vi "ResultsDB Select data.vi"(7 "CMD":T1(ring), 8 "error in (no error)":errorcluster, 9 "ItemsID":string, 11 "MainBarcode":string) -> (0 "error out":errorcluster, 2 "File Paht":string[](array[string]), 3 "30 rows":string[][](array[string]))   [LabVIEW 2015]
doc: "开始测试时根据条目自动创建条目条目，生产文件路径。\n#2020-6-8 13:25:45"
uses:
  SQLite.lvclass
  <userlib>/LabSQL/LabSQL.lvlib
  <userlib>/sushu/sushu.lvlib
  vi.lib/TopPath.lvlib
panel:
  out "32bit integer":i32
  out "size(s)":i32
  out "String":string
  out "Update CMD":string
  out "element":string
  out "Table Control":string[][](table)
  out "resulting string":string
  out "CMD":string
  out "error out 2":errorcluster
  out "match substring":string
  out "number (0 to 1)":dbl
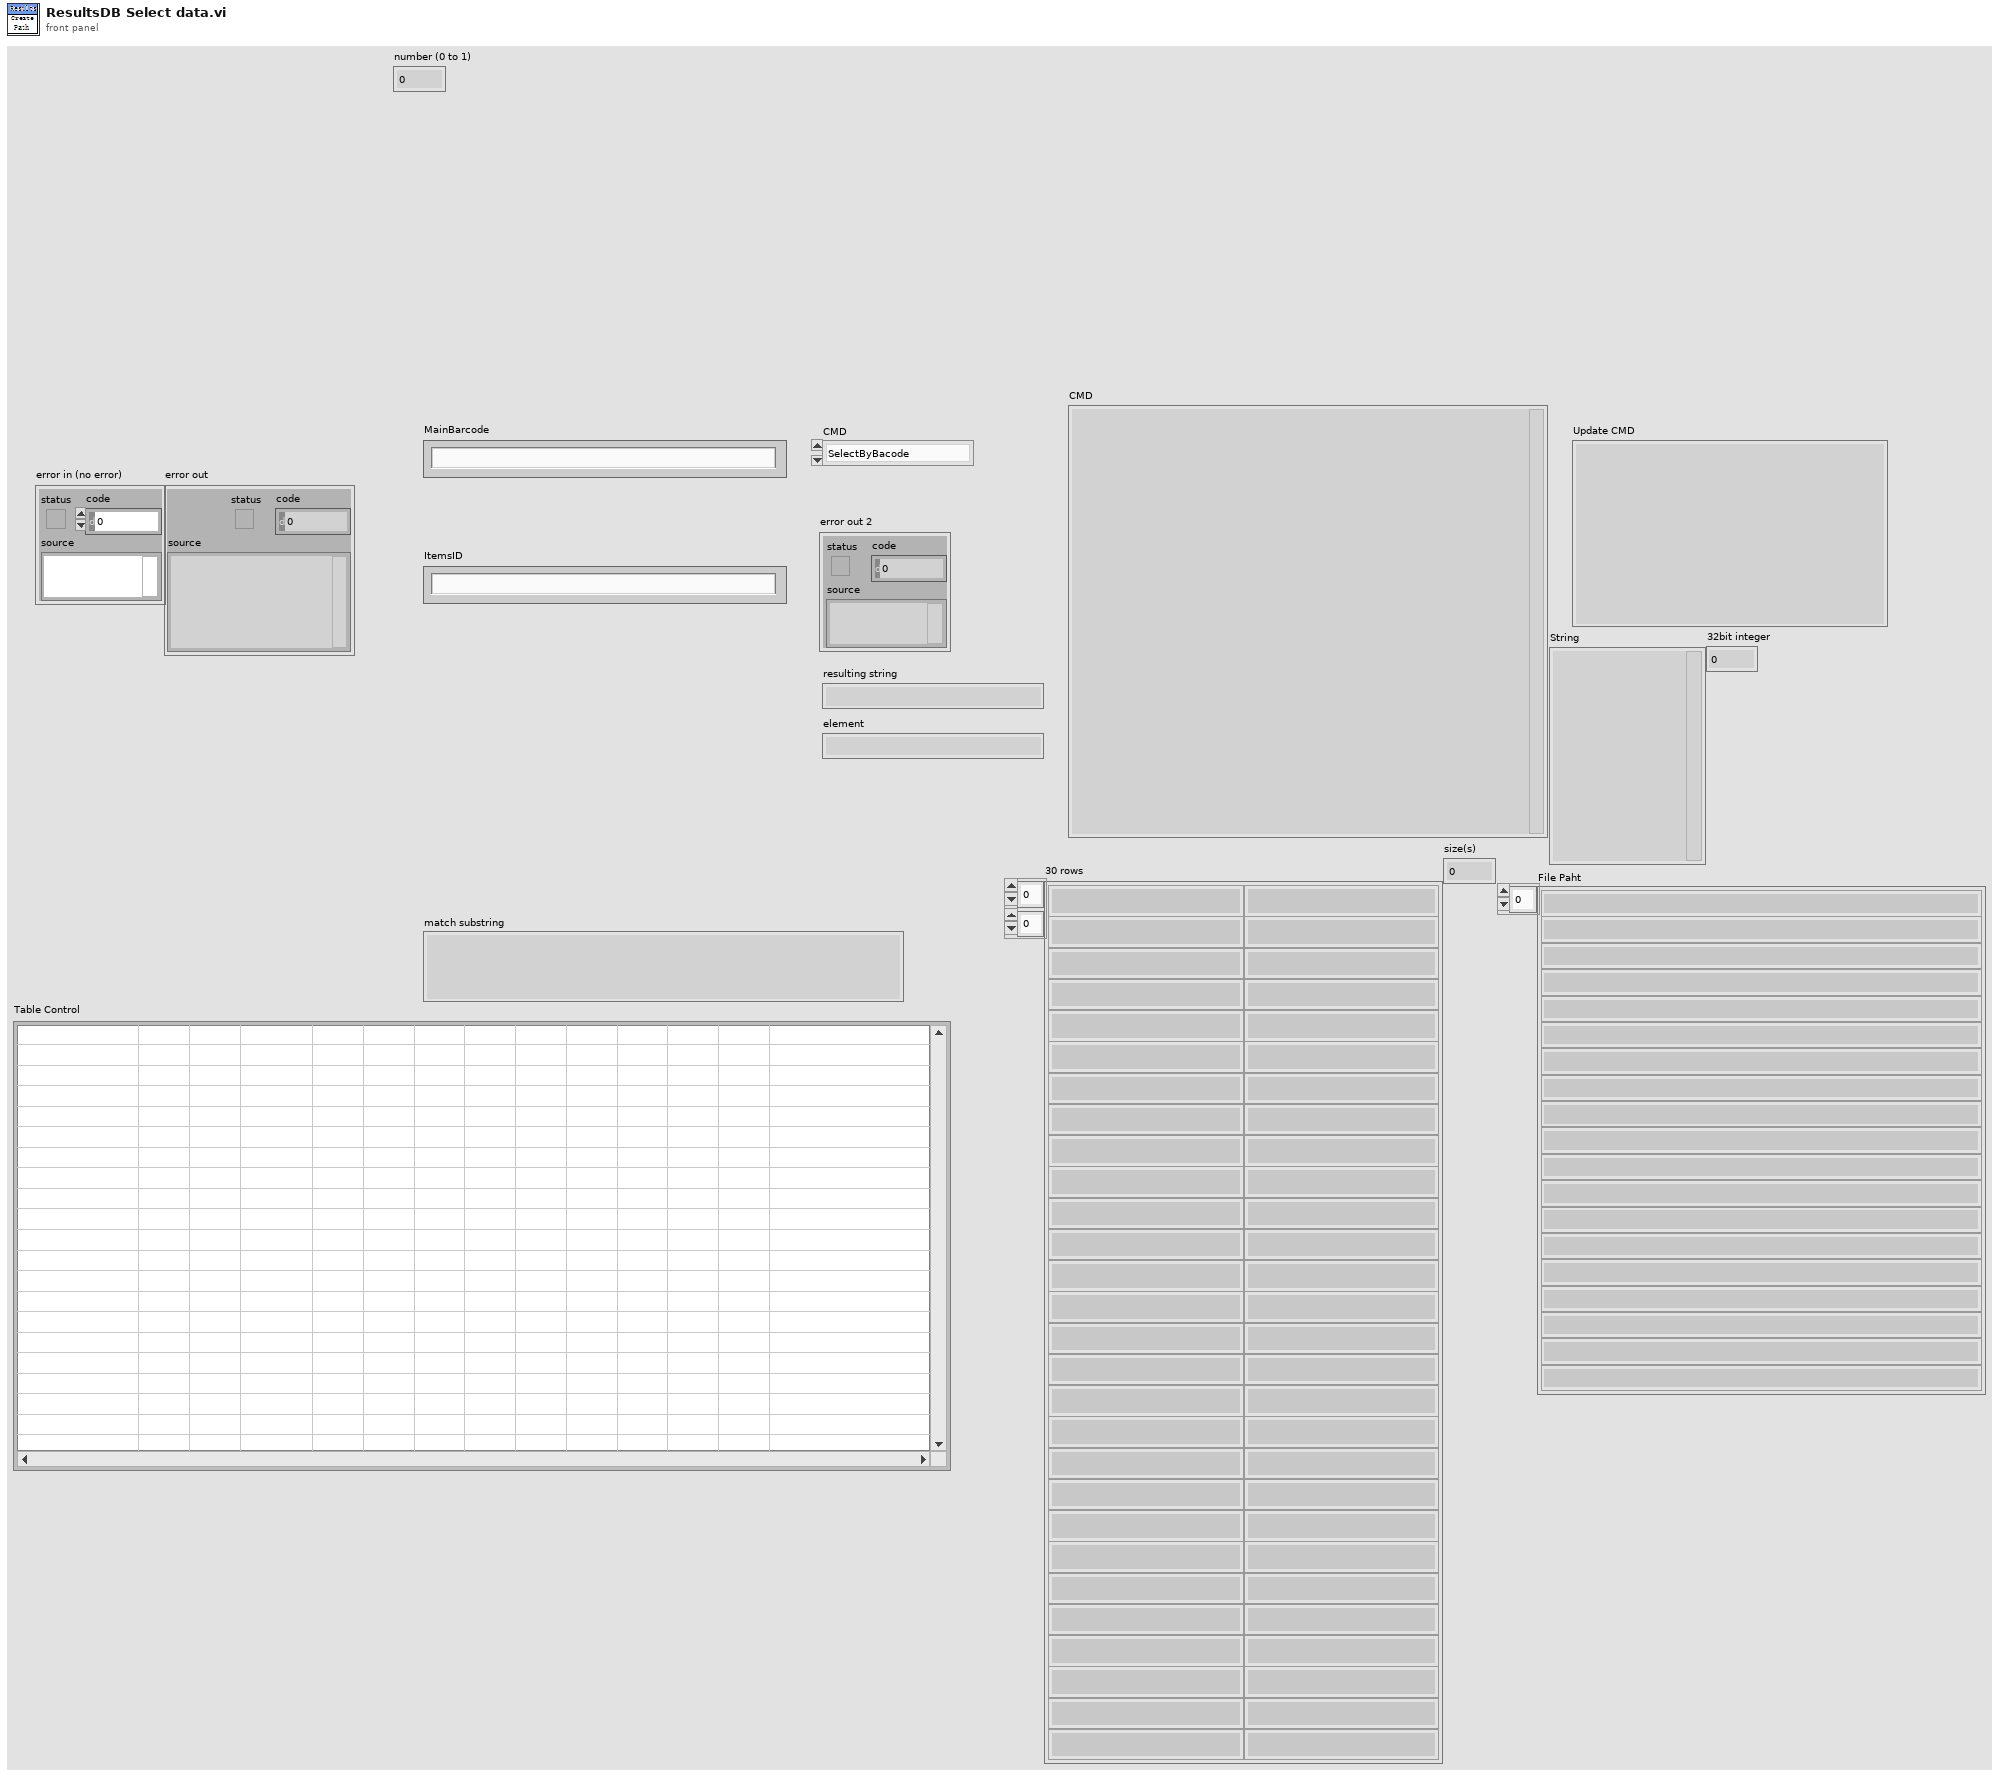
[diagram p1: front panel]
types:
  T1 = enum16{"SelectByBacode", "SelectByDatetime", "Update-UploadColumn"}
  T2 = cluster{"Core":cluster{"Current VI Reference":refnum<vi>, "Close Panel on Exit?":bool}, "VI Name":string, "Row Numbers":string, "Update?":bool, "Results Folder path":path, "CMD":string, "RowNum":i32, "ResultFilePath":path, "InsertTimes":i32}
  T3 = typedef "sushu_vi_lib.lvlib/TopPath.lvlib/Top Path.ctl" = cluster{"LV Source":path, "FilePath":path, "Data":path}
  T4 = enum16{"Other", "SQL2008", "SQLite", "Access", "MySQL"}
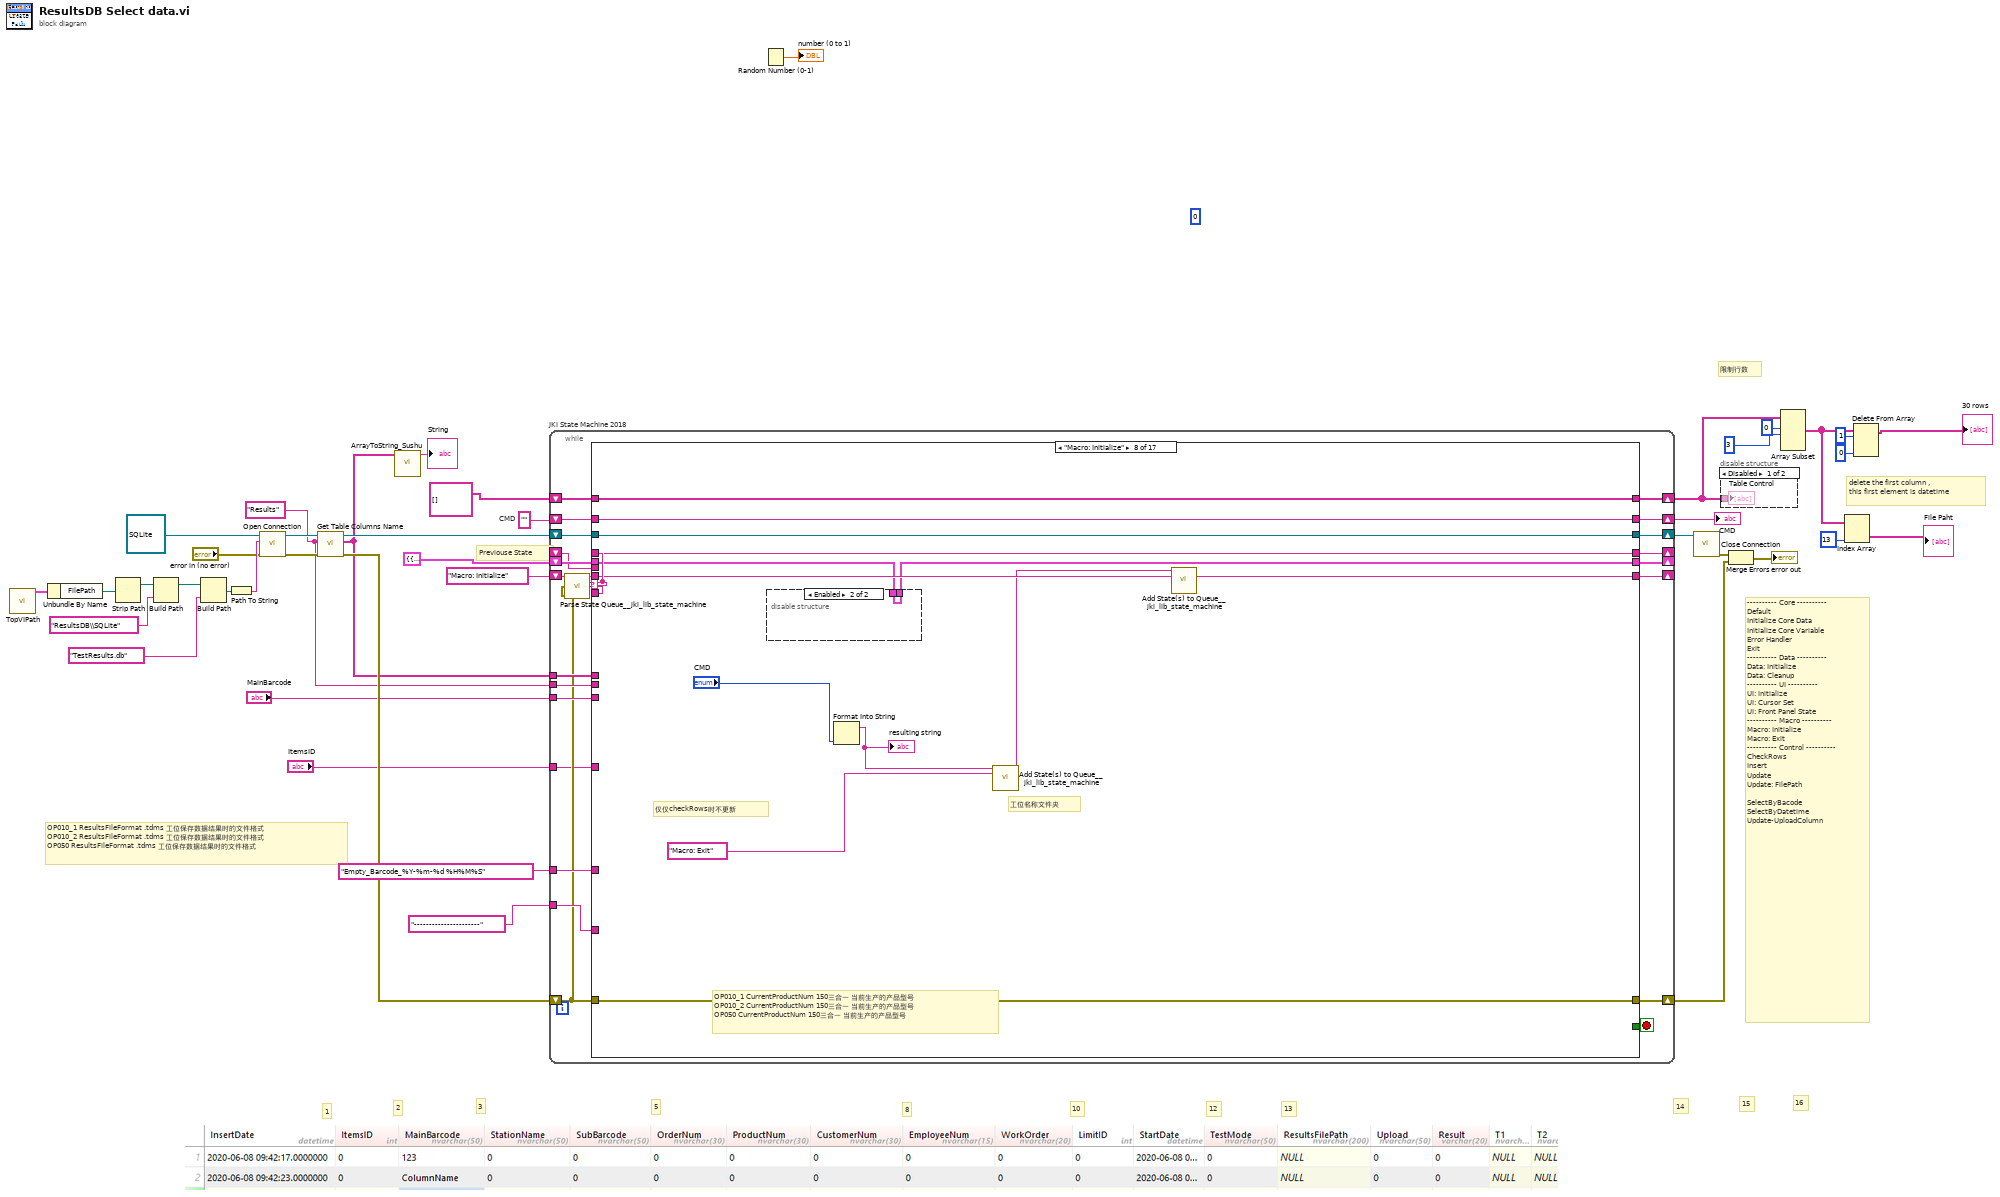
[diagram p0: block diagram]
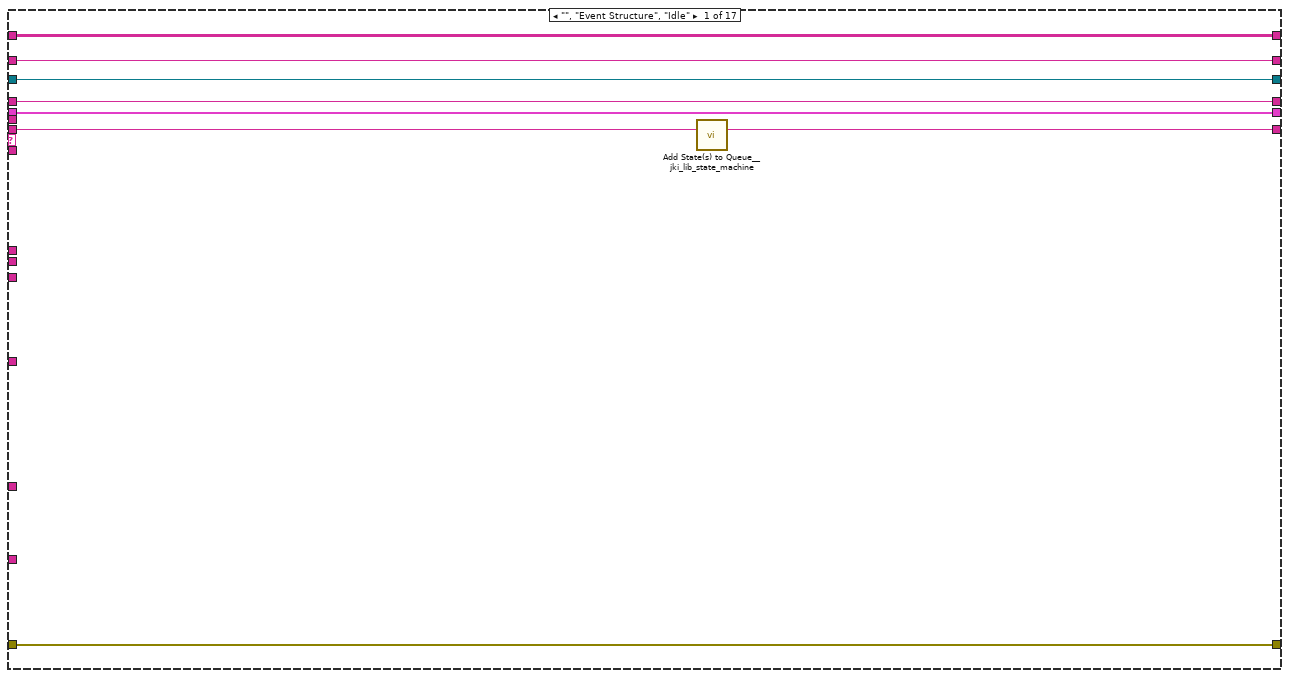
[diagram p3: hidden frame]
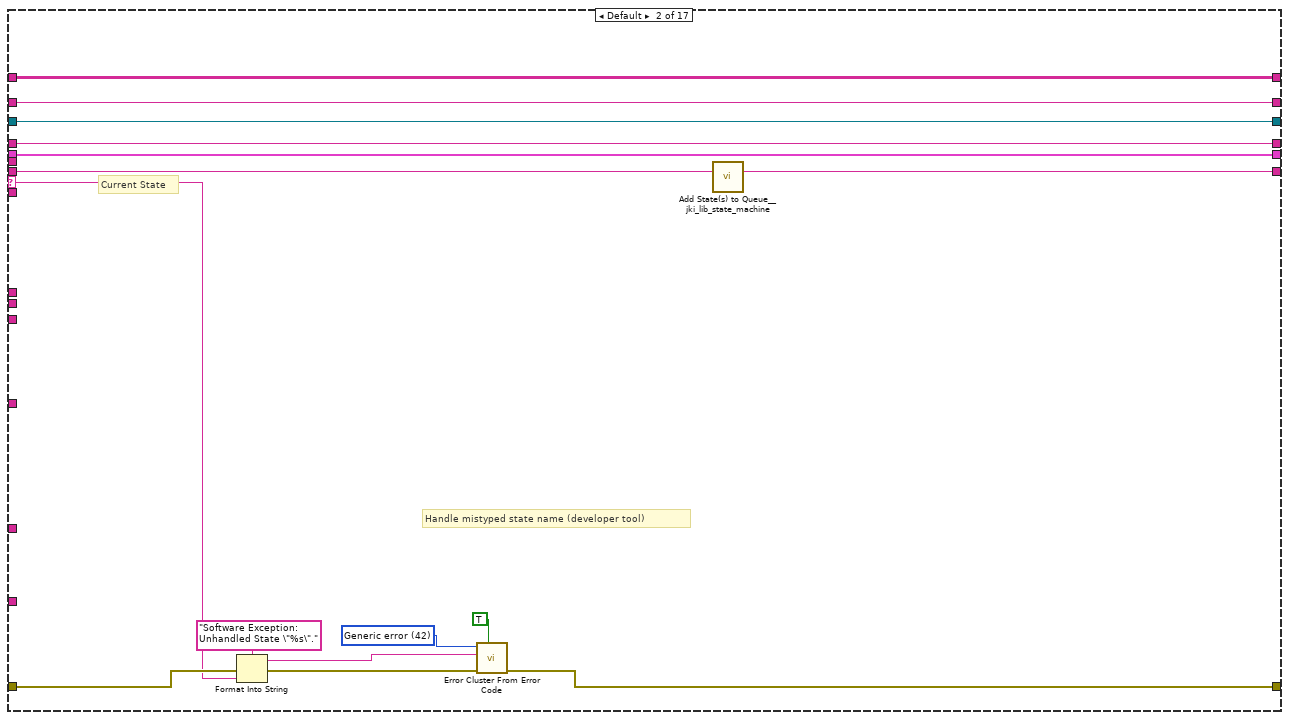
[diagram p4: hidden frame]
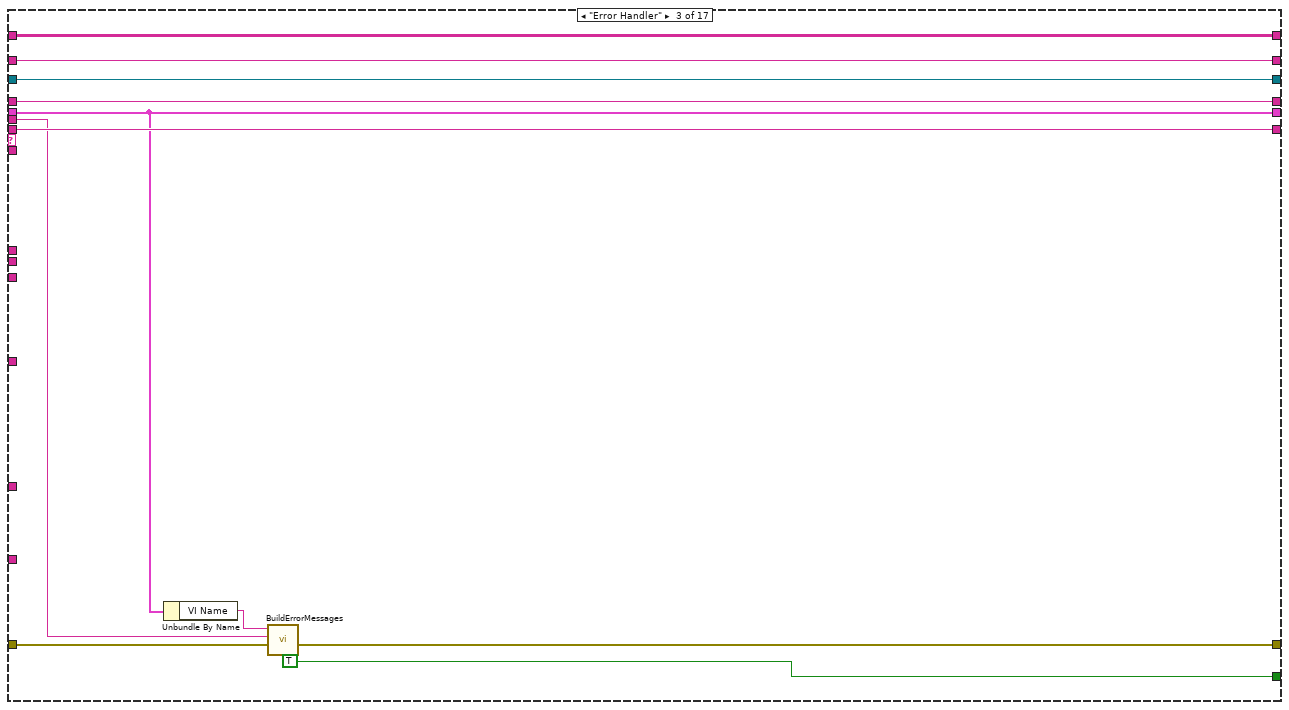
[diagram p5: hidden frame]
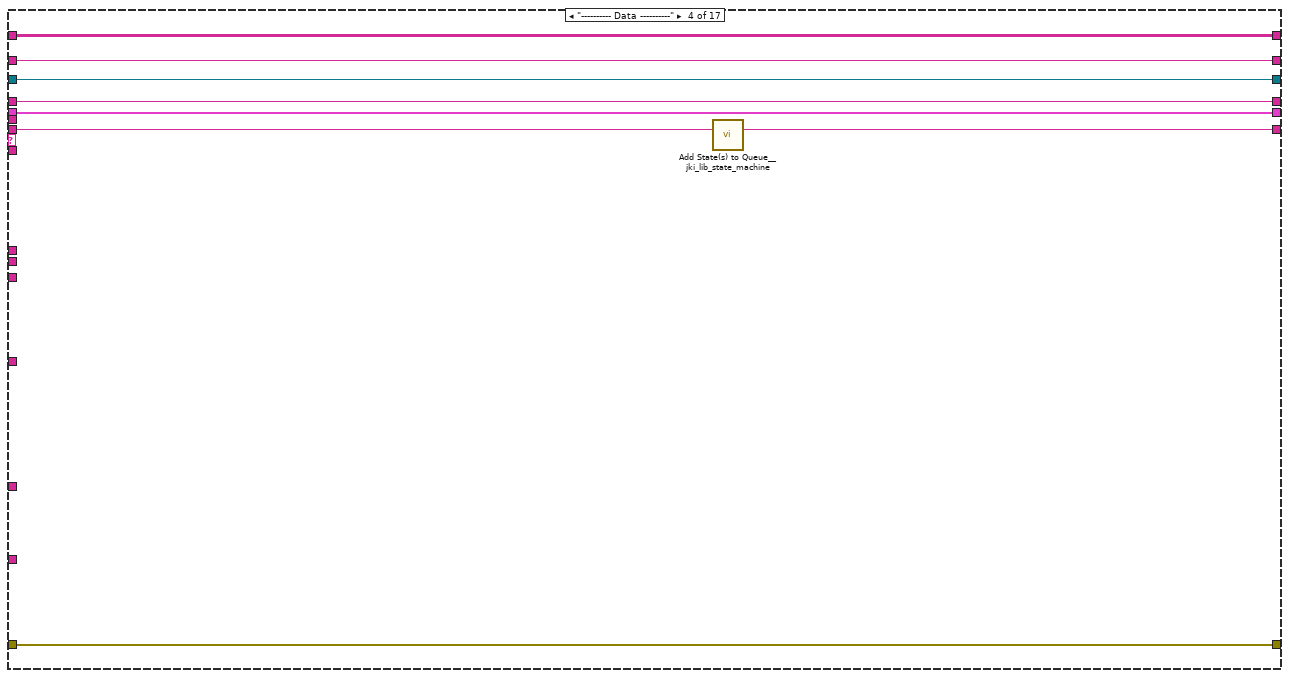
[diagram p6: hidden frame]
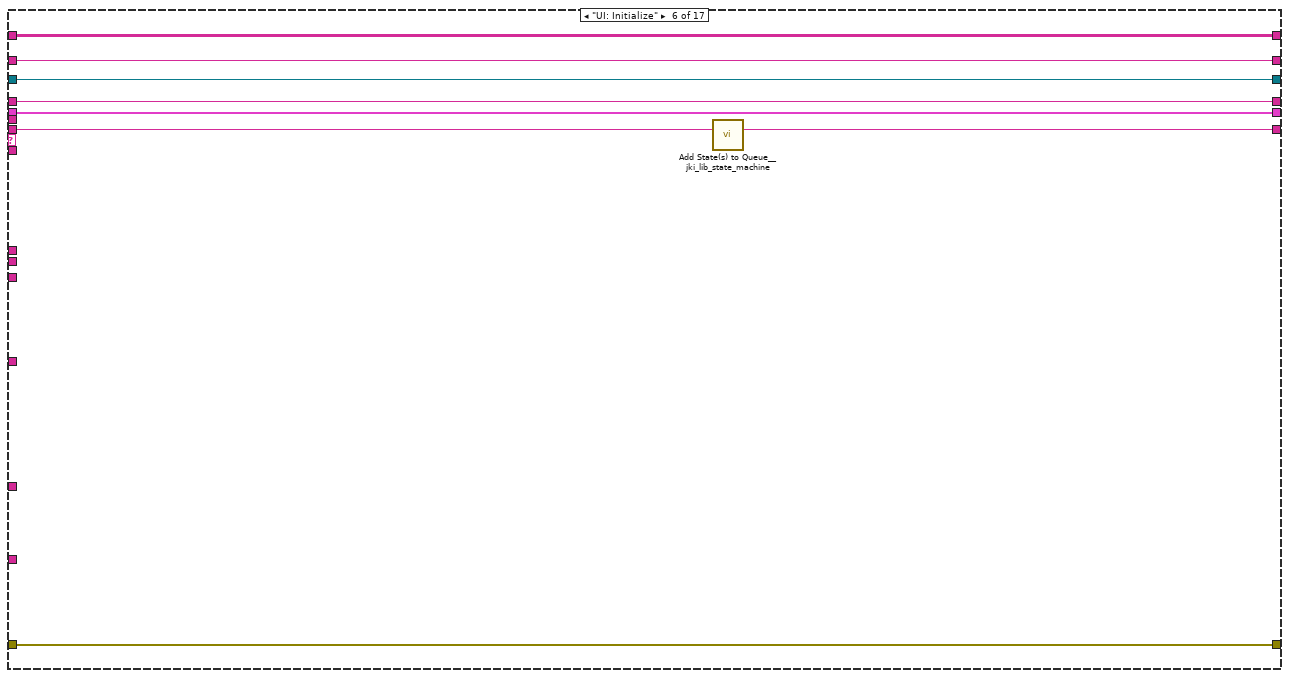
[diagram p8: hidden frame]
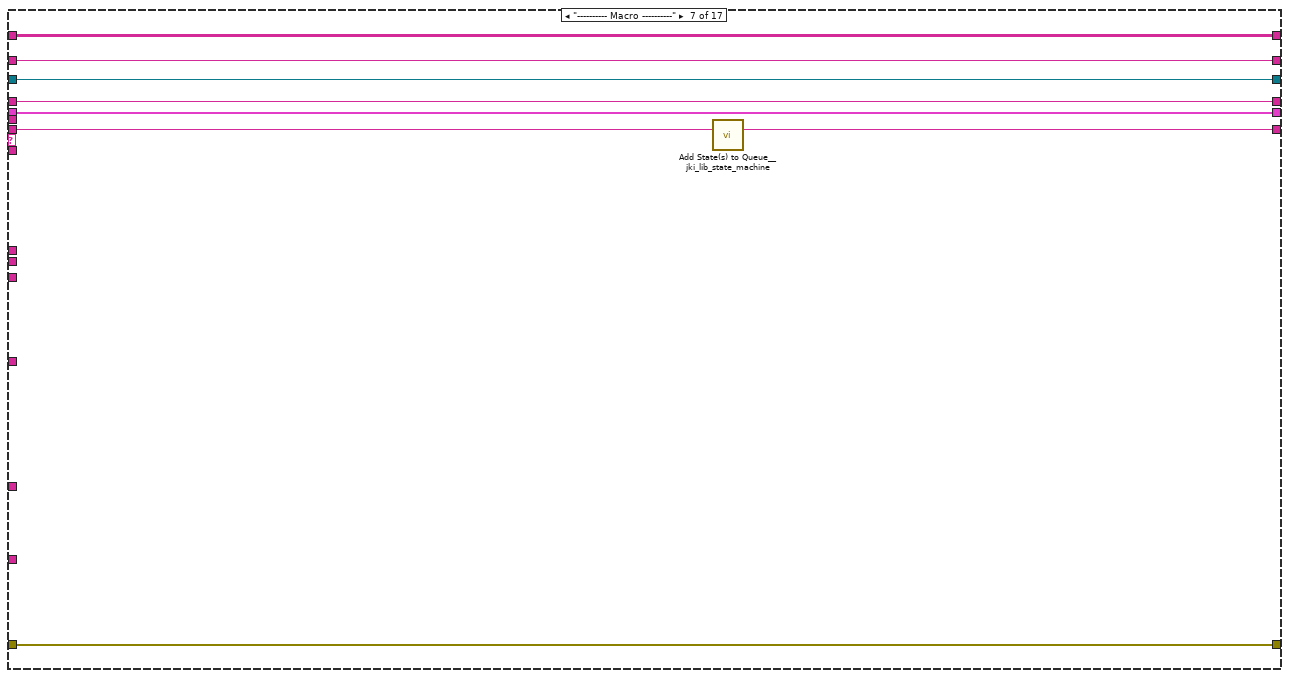
[diagram p9: hidden frame]
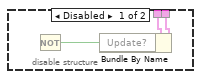
[diagram p10: hidden frame]
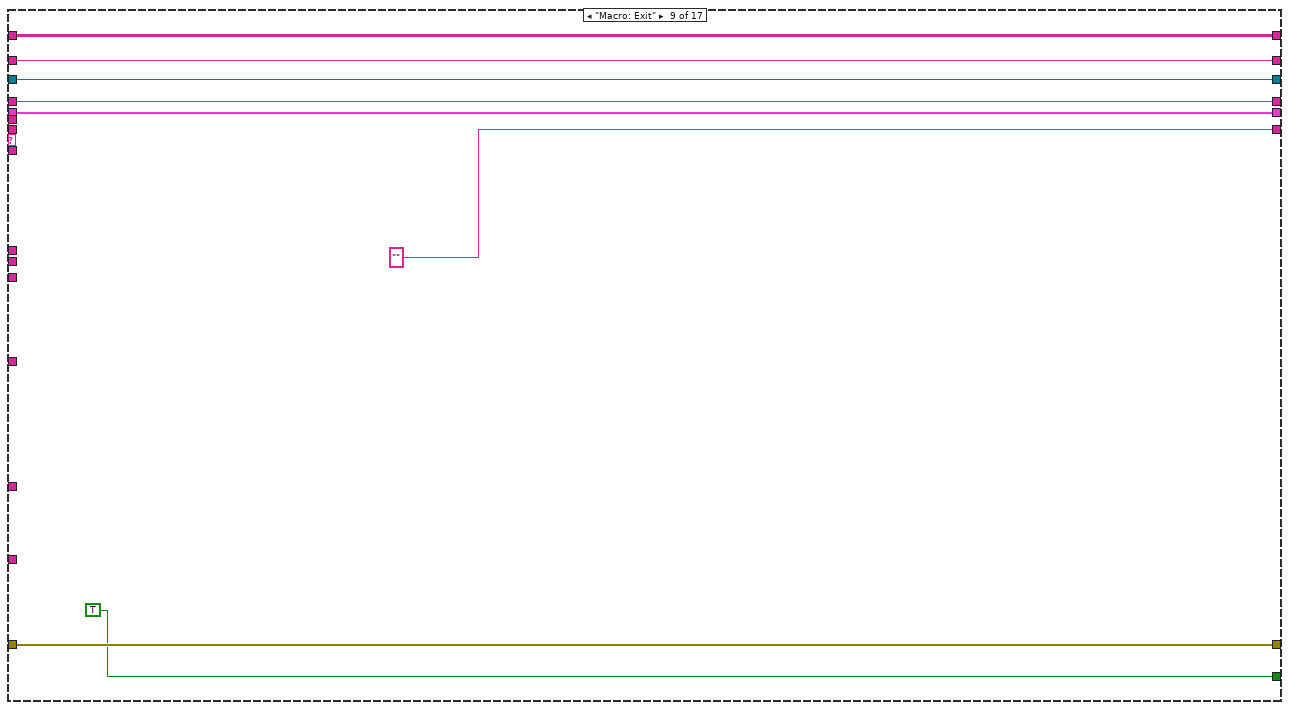
[diagram p11: hidden frame]
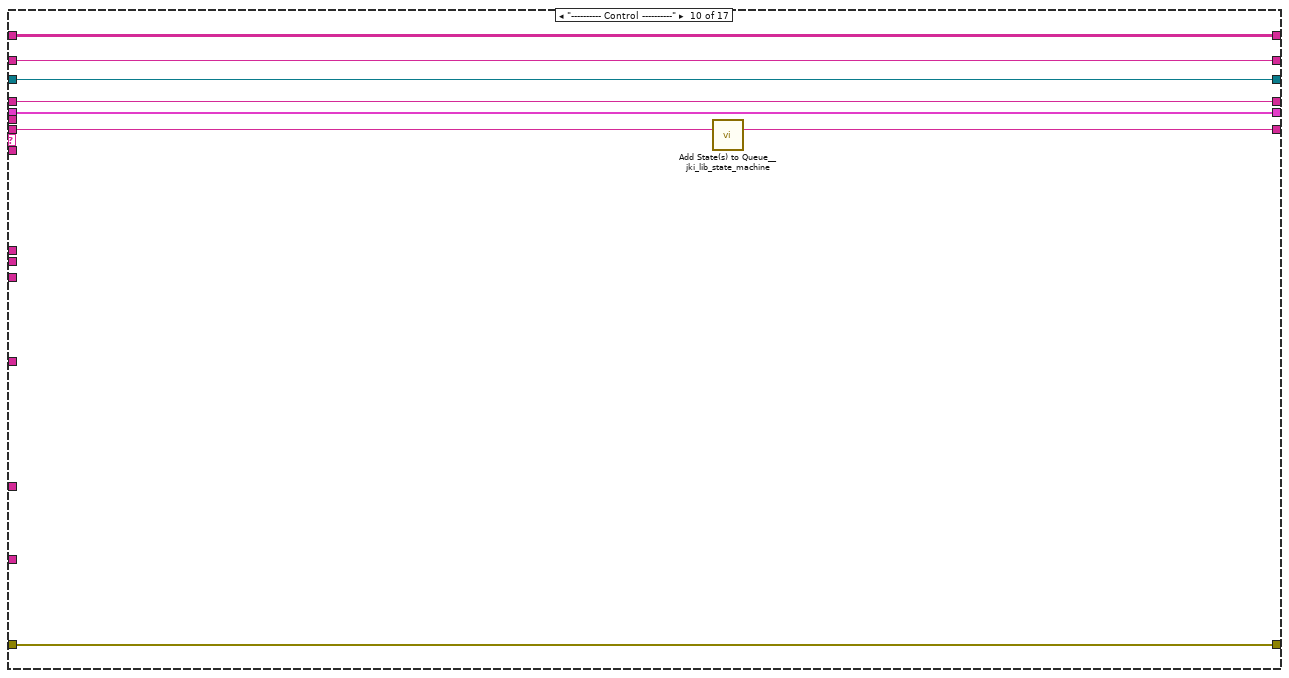
[diagram p12: hidden frame]
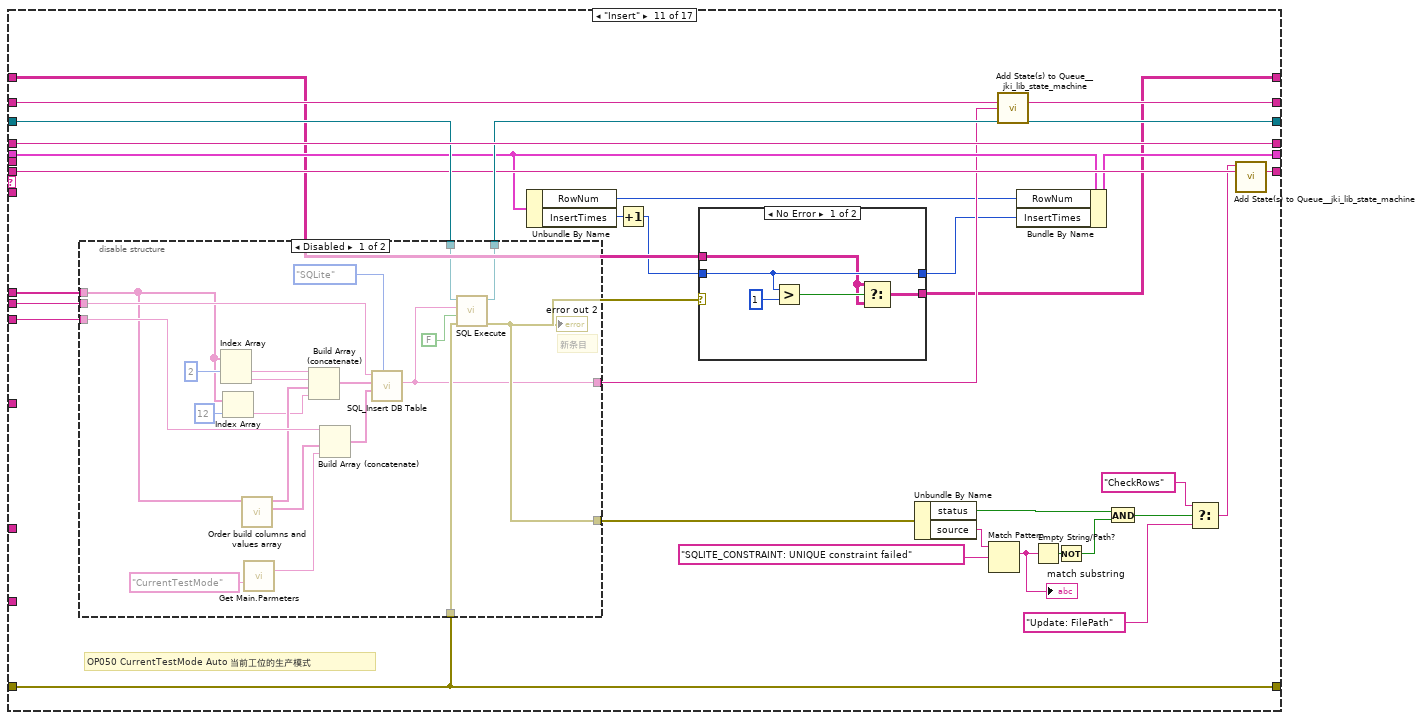
[diagram p13: hidden frame]
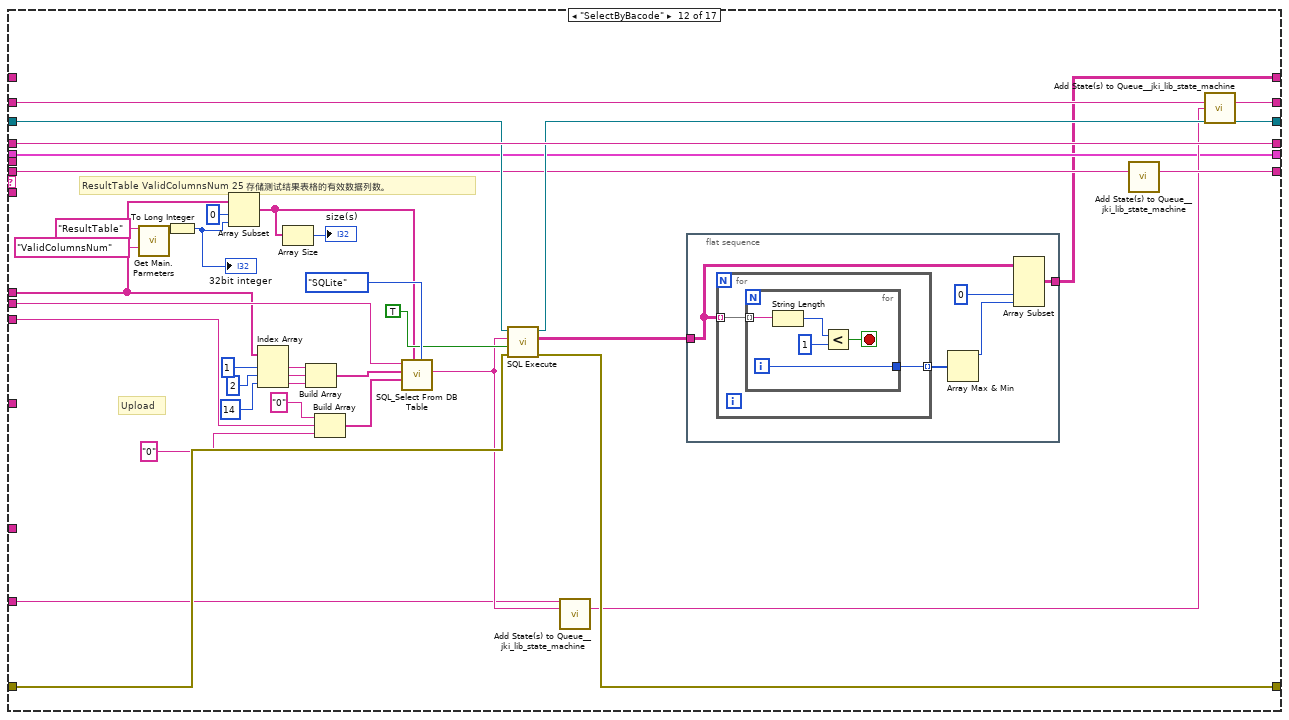
[diagram p16: hidden frame]
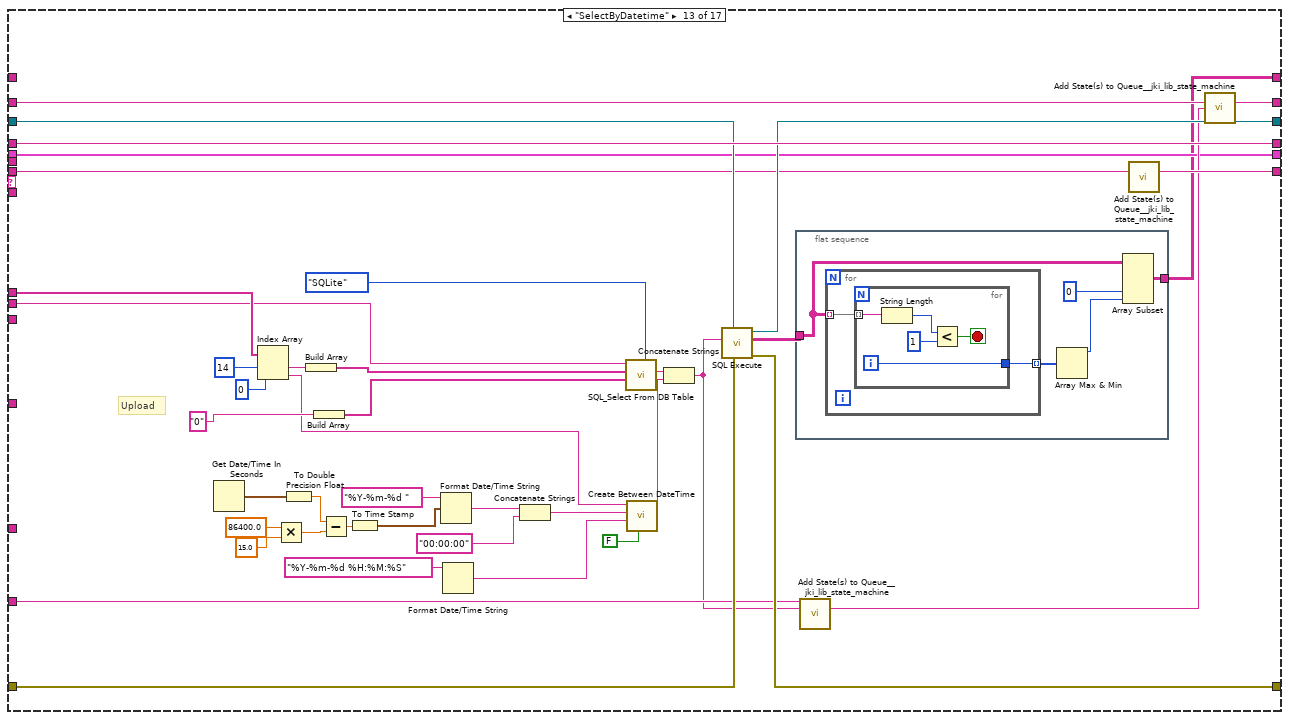
[diagram p17: hidden frame]
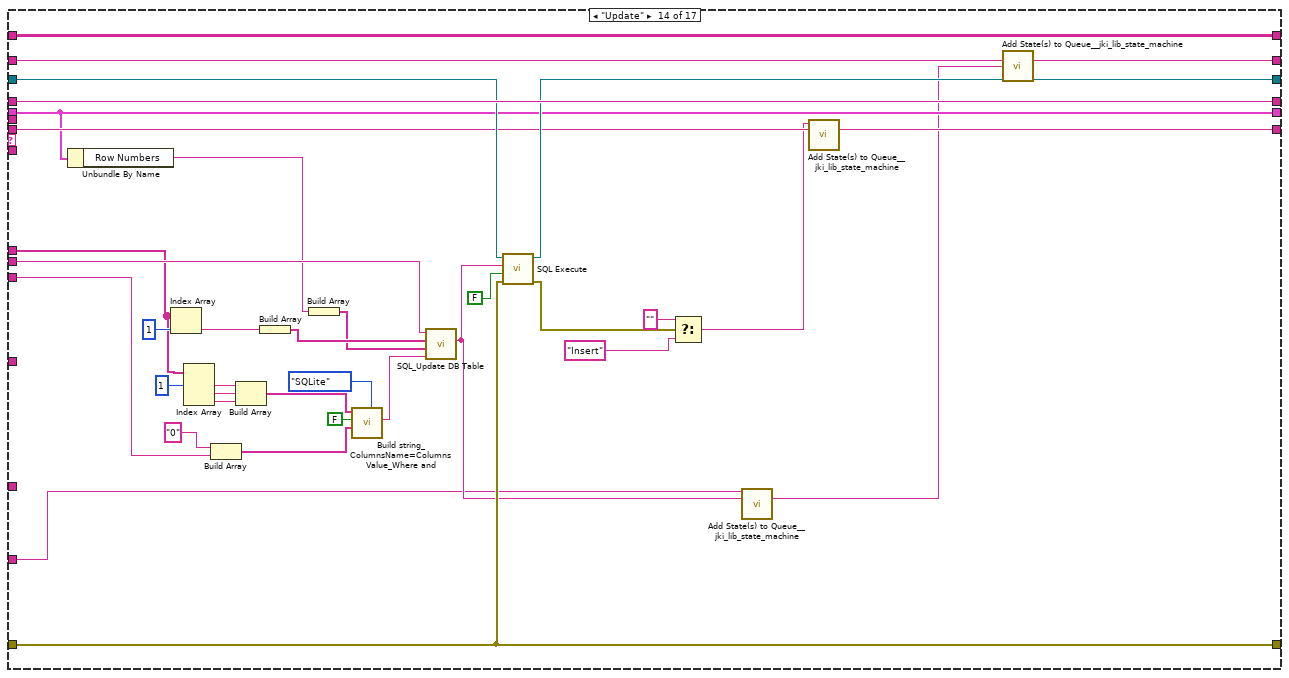
[diagram p18: hidden frame]
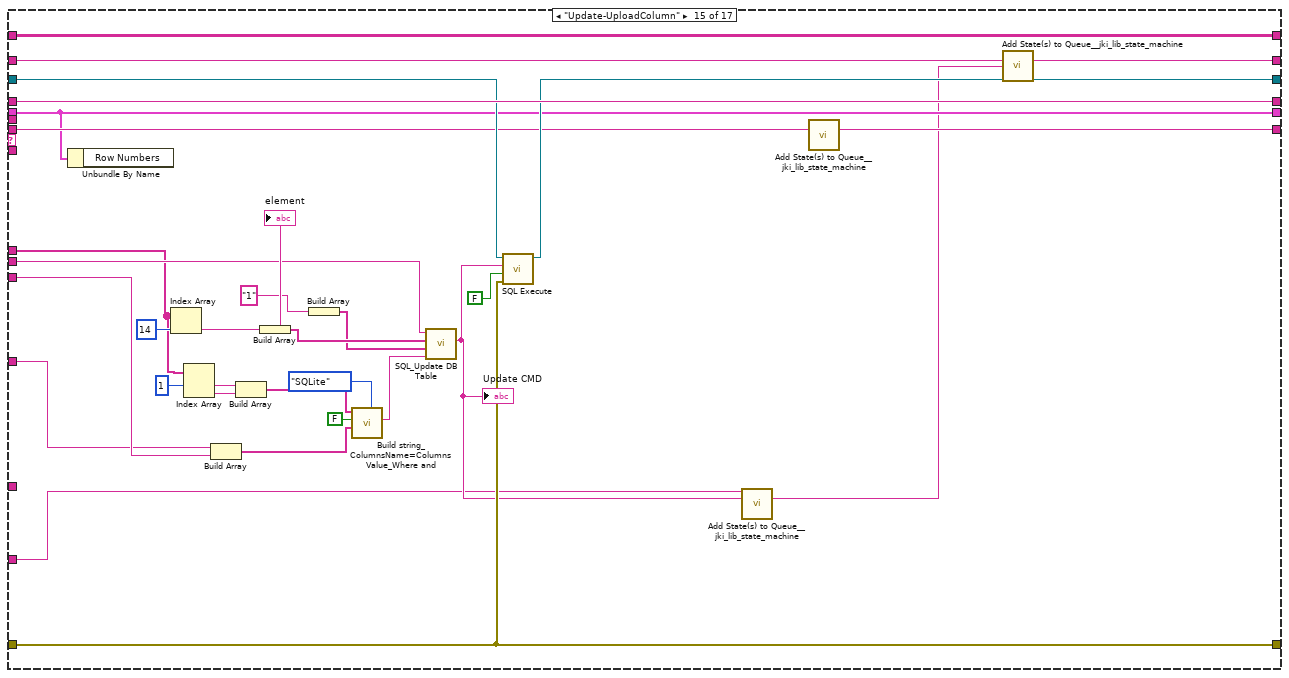
[diagram p19: hidden frame]
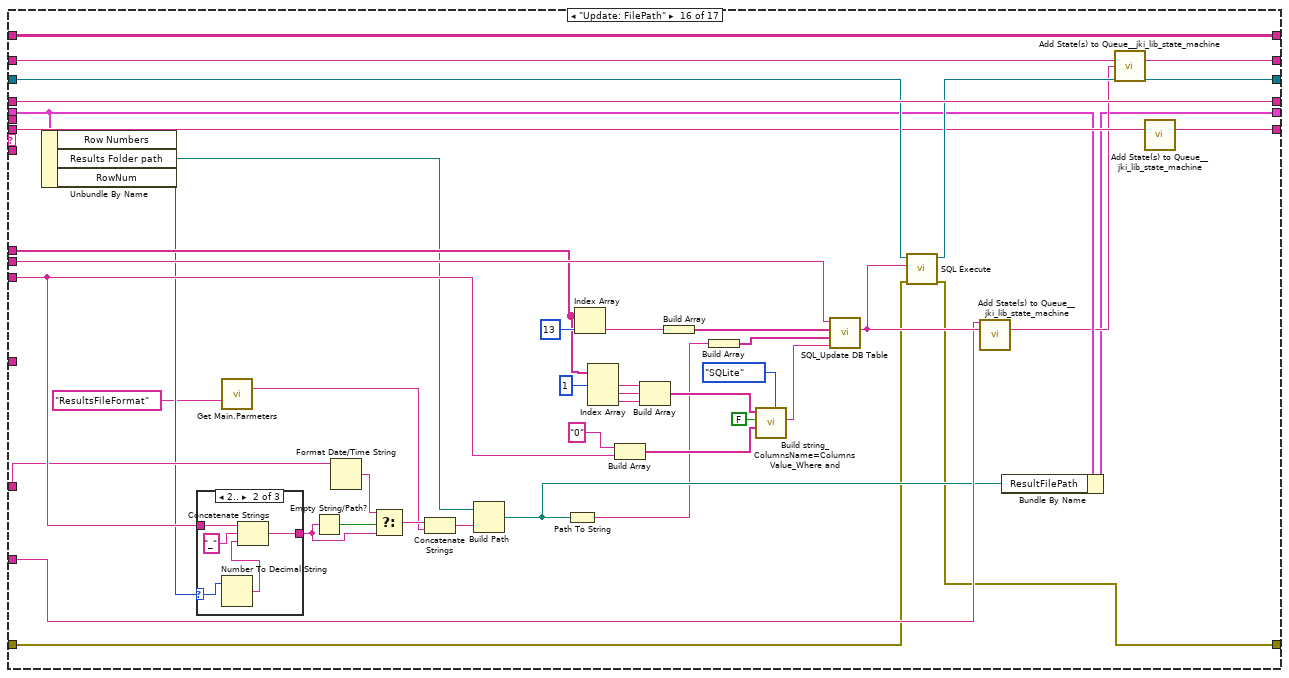
[diagram p20: hidden frame]
diagram:
  w13 = ""  # CMD
  (unwired) 0 ("index (row)")
  w19 = "Results" ("TableName")
  # "delete the first column ,\nthis first element is datetime"
  # "限制行数"
  # "OP010_1\tResultsFileFormat\t.tdms\t工位保存数据结果时的文件格式\nOP010_2\tResultsFileFormat\t.tdms\t工位保存数据结果时的文件格式\nOP050\tResultsFileFormat\t.tdms\t工位保存数据结果时的文件格式"
  # "16"
  # "15"
  # "14"
  # "13"
  # "12"
  # "10"
  # "8"
  # "5"
  # "3"
  # "2"
  # "1"
  # "Previouse State"
  # "---------- Core ----------\nDefault\nInitialize Core Data\nInitialize Core Variable\nError Handler\nExit\n---------- Data ----------\nData: Initialize\nData: Cleanup\n---------- UI ----------\nUI: Initialize\nUI: Cursor Set\nUI: Front Panel State\n---------- Macro ----------\nMacro: Initialize\nMacro: Exit\n---------- Control ----------\nCheckRows\nInsert\nUpdate\nUpdate: FilePath\n\nSelectByBacode\nSelectByDatetime\nUpdate-UploadColumn"
  n1 = call "TopVIPath.vi"() -> ("TopPath"=w27:T3)  [unwired: 10 in, 1 out]
  n2 = Unbundle By Name(w27) -> ("FilePath"=w39:path)
  n3 = Strip Path(path=w39) -> (stripped path=w38:path)  [unwired: 1 out]
  n4 = Build Path(base path=w38, name or relative path="ResultsDB\\SQLite") -> (appended path=w36:path)
  n5 = Build Path(base path=w36, name or relative path="TestResults.db") -> (appended path=w34:path)
  n6 = Path To String(path=w34) -> (string=w33:string)
  n7 = call-dynamic "Open Connection.vi"("error in (no error)"="error in (no error)", "ConnectionString"=w33, "HostDB in"=refnum<class "SQLite.lvclass"> refnum ("SQLite.lvclass")) -> ("error out"=w30:errorcluster, "HostDB out"=w31:refnum<class "SQLite.lvclass">)  [unwired: 7 in]
  n8 = call-dynamic "Get Table Columns Name.vi"("error in (no error)"=w30, "TableName"=w19, "HostDB in"=w31) -> ("error out"=w20:errorcluster, "ColunmsList"=w2:string[], "HostDB out"=w24:refnum<class "SQLite.lvclass">)  [unwired: 4 in, 2 out]
  n9 = call <userlib>:"ArrayToString_Sushu.vi"("Array"=w2) -> ("String"=→"String":string)  [unwired: 10 in]
  n10 = while "JKI State Machine 2018" {
    shift-right: [w58] -> _
    shift-left: T2 {"Core"={"Current VI Reference"=refnum, "Close Panel on Exit?"=FALSE}, "VI Name"="", "Row Numbers"="", "Update?"=FALSE, "Results Folder path"=path "", "CMD"="", "RowNum"=0, "ResultFilePath"=path "", "InsertTimes"=0} ("Data") -> [w57]
    shift-right: [w61] -> w21
    shift-left: w20 -> [w42]
    shift-right: [w60] -> _
    shift-left: "Macro: Initialize" -> [w62]
    shift-right: [w55] -> w23
    shift-left: w24 -> [w56]
    shift-right: [w53] -> _
    shift-left: _ -> [w52]
    tunnel: "MainBarcode" -> [w51]
    tunnel: w2 -> [w50]
    tunnel: w19 -> [w49]
    tunnel: "Empty_Barcode_%Y-%m-%d %H%M%S" ("time format string (%c)") -> [w48]
    shift-right: [w47] -> w15
    shift-left: w13 -> [w46]
    tunnel: "----------------------" ("State(s) in (\"\")") -> [w45]
    shift-right: [w43] -> w10
    shift-left: string[][] [] ("Table Control") -> [w44]
    tunnel: "ItemsID" -> [w41]
    stop <- w59 stop-if-true
    n11 = call <vilib>:"Parse State Queue__jki_lib_state_machine.vi"("State Queue"=w62, "Error In (no error)"=w42) -> ("Remaining States"=w64:string, "Current State"=w54:string, "Arguments"=w63:string)  [unwired: 11 in]
    n12 = case shown="\"Macro: Initialize\"" w54 {
      selector: w54 -> [_ w77 _ _ _ _ _ _ _ _ _ _ _ _ _ _ _]
      tunnel: w64 -> [w72 w81 w97 w106 w110 w121 w129 w142 _ w162 w178 w247 w300 w348 w379 w426 w448]
      tunnel: w63 -> [_ _ _ _ _ _ _ _ _ _ _ _ _ _ _ _ _]
      tunnel: w57 -> [w69 w79 w94 w103 w111 w119 w126 w137 w153 w159 w175 w239 w292 w347 w378 w405 w447]
      tunnel: [w70 w83 w90 w104 w113 w118 w127 w138 w154 w160 w188 w245 w298 w350 w381 w391 w449] -> w61
      tunnel: w42 -> [w70 w82 w91 w104 w113 w118 w127 w138 w154 w160 w188 w246 w299 w350 w381 w393 w449]
      tunnel: [w71 w80 w97 w105 w110 w120 w128 w141 "" w161 w179 w248 w301 w349 w380 w427 w448] -> w60
      tunnel: [_ _ TRUE _ _ _ _ _ TRUE _ _ _ _ _ _ _ _] -> w59
      tunnel: [w69 w79 w94 w103 w111 w119 w126 w132 w153 w159 w174 w239 w292 w347 w378 w398 w447] -> w58
      tunnel: w56 -> [w68 w76 w96 w102 w112 w117 w125 w140 w152 w158 w190 w251 w303 w353 w384 w429 w446]
      tunnel: [w68 w76 w96 w102 w112 w117 w125 w140 w152 w158 w189 w250 w302 w352 w383 w428 w446] -> w55
      tunnel: w54 -> [w67 w75 w95 w101 w109 w116 w124 w139 w150 w157 w193 w258 w311 w359 w390 w434 w445]
      tunnel: [w67 w75 w95 w101 w109 w116 w124 w139 w150 w157 w193 w258 w311 w359 w390 w434 w445] -> w53
      tunnel: w52 -> [_ _ w92 _ _ _ _ _ _ _ _ _ _ _ _ _ _]
      tunnel: w51 -> [_ _ _ _ _ _ _ _ _ _ w191 w252 _ w354 w385 w408 _]
      tunnel: w50 -> [_ _ _ _ _ _ _ _ _ _ w169 w233 w305 w342 w374 w422 _]
      tunnel: w49 -> [_ _ _ _ _ _ _ _ _ _ w192 w253 w304 w355 w386 w430 _]
      tunnel: w48 -> [_ _ _ _ _ _ _ _ _ _ _ _ _ _ _ w407 _]
      tunnel: w46 -> [w66 w74 w89 w100 w108 w115 w123 w134 w148 w156 w173 w243 w296 w328 w366 w403 w444]
      tunnel: [w66 w74 w89 w100 w108 w115 w123 w134 w148 w156 w172 w244 w297 w329 w367 w404 w444] -> w47
      tunnel: w45 -> [_ _ _ _ _ _ _ _ _ _ _ w240 w293 w325 w363 w400 _]
      tunnel: w44 -> [w65 w73 w88 w99 w107 w114 w122 w133 w147 w155 w167 _ _ w324 w362 w392 w443]
      tunnel: [w65 w73 w88 w99 w107 w114 w122 w133 w147 w155 w166 w234 w271 w324 w362 w392 w443] -> w43
      tunnel: w41 -> [_ _ _ _ _ _ _ _ _ _ _ _ _ _ w360 _ _]
      frame "", "Event Structure", "Idle" {
        n13 = call <vilib>:"Add State(s) to Queue__jki_lib_state_machine.vi"("State(s) in (\"\")"=w72) -> ("States Out"=w71:string)  [unwired: 14 in]
      }
      frame Default {
        w86 = 42 items=["No error", "Argument error", "Memory is full", "Out of zone", "End of file", "File already open", "Generic file I/O error", "File not found", "File permission error", "Disk is full", "Duplicate path", "Too many files open", "System feature not enabled", "Resource file not found", "Cannot add resource", "Resource not found", "Image not found", "Image memory error", "Pen does not exist", "Config type invalid", "Config token not found", "Config parse error", "Config memory error", "Bad external code format", "Bad external code offset", "External code not present", "Null window", "Destroy window error", "Null menu", "Print aborted", "Bad print record", "Print driver error", "Windows error during printing", "Memory error during printing", "Print dialog error", "Generic print error", "Invalid device refnum", "Device not found", "Device parameter error", "Device unit error", "Cannot open device", "Device call aborted", "Generic error", "Cancelled by user", "Object ID too low", "Object ID too high", "Object not in heap", "Unknown heap", "Unknown object (invalid DefProc)", "Unknown object (DefProc not in table)", "Message out of range", "Invalid (null) method", "Unknown message", "Manager call not supported", "Bad address", "Network operation in progress", "Network operation timed out", "Connection is busy", "Network attribute not supported", "Network error", "Address in use", "System out of memory", "Connection aborted", "Connection refused", "Not connected", "Already connected", "Connection closed", "Initialization error (interapplication manager)", "Bad occurrence", "Wait on unbound occurrence handler", "Occurrence queue overflow", "Datalog type conflict", "Unused", "Unrecognized type (interapplication manager)", "Memory corrupt", "Failed to make temporary DLL", "Old CIN version", "Drag socket not found", "Failed to load drop-object", "Failed to register OLE object", "Failed to release OLE object", "Format specifier type mismatch", "Unknown format specifier", "Too few format specifiers", "Too many format specifiers", "Scan failed", "Newer CIN version", "Error converting to variant", "Runtime menu error", "Password tampered", "Variant attribute not found", "Incompatible variant data type", "Event data is not available", "Event Store is not present", "Occurrence is not found", "Event Queue is not created", "Event info is not available", "Refnum passed is NULL", "Error retrieving Class GUID", "Error retrieving CoClass GUID", "Error retrieving TypeLib GUID.", "Bad built application magic bytes.", "Specific driver is different from the specific driver associated with the Logical Name.", "There is no session opened to the class driver.", "Max Error", "MAX - Error with config objects", "MAX - Error loading configuration", "MAX - Group not supported"]
        # "Current State"
        # "Handle mistyped state name (developer tool)"
        n14 = Format Into String(format string="Software Exception: Unhandled State \"%s\"." ("message"), error in=w82, w77) -> (resulting string=w85:string, error out=w84:errorcluster)  [unwired: 1 in]
        n15 = call <vilib>:"Error Cluster From Error Code.vi"("show call chain? (False)"=TRUE, "error in (no error)"=w84, "error message (\"\")"=w85, "error code (0)"=w86) -> ("error out"=w83:errorcluster)  [unwired: 5 in]
        n16 = call <vilib>:"Add State(s) to Queue__jki_lib_state_machine.vi"("State(s) in (\"\")"=w81) -> ("States Out"=w80:string)  [unwired: 14 in]
      }
      frame "Error Handler" {
        n17 = Unbundle By Name(w94) -> ("VI Name"=w93:string)
        n18 = call <userlib>:"BuildErrorMessages.vi"("error in"=w91, "ErrorCase"=w92, "VI Name"=w93) -> ("error out (no error)"=w90:errorcluster)  [unwired: 6 in, 2 out]
      }
      frame "---------- Data ----------" {
        n19 = call <vilib>:"Add State(s) to Queue__jki_lib_state_machine.vi"("State(s) in (\"\")"=w106) -> ("States Out"=w105:string)  [unwired: 14 in]
      }
      frame "Data: Initialize" {
      }
      frame "UI: Initialize" {
        n20 = call <vilib>:"Add State(s) to Queue__jki_lib_state_machine.vi"("State(s) in (\"\")"=w121) -> ("States Out"=w120:string)  [unwired: 14 in]
      }
      frame "---------- Macro ----------" {
        n21 = call <vilib>:"Add State(s) to Queue__jki_lib_state_machine.vi"("State(s) in (\"\")"=w129) -> ("States Out"=w128:string)  [unwired: 14 in]
      }
      frame "Macro: Initialize" {
        # "OP010_1\tCurrentProductNum\t150三合一\t当前生产的产品型号\nOP010_2\tCurrentProductNum\t150三合一\t当前生产的产品型号\nOP050\tCurrentProductNum\t150三合一\t当前生产的产品型号"
        # "工位名称文件夹"
        # "仅仅checkRows时不更新"
        n22 = disable-structure shown="Enabled" {
          disable-tunnel: w137 -> [w145 w146]
          disable-tunnel: [w144 w146] -> w132
          frame Disabled {
            n23 = Not() -> (.not. x?=w143:bool)  [unwired: 1 in]
            n24 = Bundle By Name(cluster=w145, "Update?"=w143) -> (w144:T2)
          }
          frame Enabled {
          }
        }
        n25 = Format Into String("CMD") -> (resulting string=w130:string)  [unwired: 3 in, 1 out]
        "resulting string" <- w130
        n26 = call <vilib>:"Add State(s) to Queue__jki_lib_state_machine.vi"("State(s) in Front (\"\")"=w130, "State(s) in (\"\")"="Macro: Exit") -> ("States Out"=w136:string)  [unwired: 13 in]
        n27 = call <vilib>:"Add State(s) to Queue__jki_lib_state_machine.vi"("State(s) in Front (\"\")"=w136, "State(s) in (\"\")"=w142) -> ("States Out"=w141:string)  [unwired: 13 in]
      }
      frame "Macro: Exit" {
      }
      frame "---------- Control ----------" {
        n28 = call <vilib>:"Add State(s) to Queue__jki_lib_state_machine.vi"("State(s) in (\"\")"=w162) -> ("States Out"=w161:string)  [unwired: 14 in]
      }
      frame "Insert" {
        # "OP050\tCurrentTestMode\tAuto\t当前工位的生产模式"
        n29 = disable-structure shown="Disabled" {
          disable-tunnel: w192 -> [w208 _]
          disable-tunnel: w191 -> [w207 _]
          disable-tunnel: w190 -> [w206 _]
          disable-tunnel: [w205 _] -> w189
          disable-tunnel: w188 -> [w203 _]
          disable-tunnel: [w200 _] -> w171
          disable-tunnel: w169 -> [w197 _]
          disable-tunnel: [w194 _] -> w168
          frame Disabled {
            # "新条目"
            n30 = Index Array(array=w197, index #1=2 ("index")) -> (element #1=w213:string, element #2=w214:string)  [unwired: 1 in]
            n31 = Index Array(array=w197, index=12) -> (element=w195:string)
            n32 = call "Order build columns and values array.vi"("ColunmsList"=w197) -> ("Order values Array"=w201:string[], "Order Columns Array"=w202:string[])  [unwired: 9 in]
            n33 = call "Get Main.Parmeters.vi"("VariableName"="CurrentTestMode") -> ("Value"=w198:string)  [unwired: 8 in, 6 out]
            n34 = Build Array (concatenate)(w213, w214, w202, w195) -> (w211:string[])
            n35 = Build Array (concatenate)(w207, w201, w198) -> (w210:string[])  [unwired: 1 in]
            n36 = call <userlib>:"SQL_Insert DB Table.vi"("DB Type"=T4."SQLite", "ColumnsValue"=w210, "ColumnsName"=w211, "Table Name"=w208) -> ("Insert DB String"=w200:string)  [unwired: 7 in]
            n37 = call-dynamic "SQL Execute.vi"("error in (no error)"=w203, "Return Data (T)"=FALSE, "Command Text"=w200, "HostDB in"=w206) -> ("error out"=w194:errorcluster, "HostDB out"=w205:refnum<class "SQLite.lvclass">)  [unwired: 3 in, 3 out]
            "error out 2" <- w194
          }
          frame Enabled {
          }
        }
        n38 = Unbundle By Name(w175) -> ("RowNum"=w170:i32, "InsertTimes"=w164:i32)
        n39 = Increment(x=w164) -> (x+1=w163:i32)
        n40 = case shown="No Error" w168 {
          tunnel: w163 -> [w216 w220]
          tunnel: w167 -> [w215 w221]
          tunnel: [w217 w221] -> w166
          tunnel: [w216 w220] -> w165
          frame No Error {
            n41 = Greater?(x=w216, y=1) -> (0:w218:bool)
            n42 = Select(t=w215, s=w218, f=w215) -> (s? t:f=w217:string[][])
          }
          frame Error {
          }
        }
        n43 = Unbundle By Name(w168) -> ("status"=w184:bool, "source"=w187:string)
        n44 = Match Pattern(string=w187, regular expression="SQLITE_CONSTRAINT: UNIQUE constraint failed") -> (match substring=w185:string)  [unwired: 1 in, 3 out]
        "match substring" <- w185
        n45 = call <vilib>:"Add State(s) to Queue__jki_lib_state_machine.vi"("State(s) in (\"\")"=w173, "State(s) at Back (\"\")"=w171) -> ("States Out"=w172:string)  [unwired: 13 in]
        n46 = Bundle By Name(cluster=w175, "RowNum"=w170, "InsertTimes"=w165) -> (w174:T2)
        n47 = Empty String/Path?(string/path=w185) -> (empty?=w183:bool)
        n48 = Not(x=w183) -> (.not. x?=w176:bool)
        n49 = And(x=w184, y=w176) -> (x .and. y?=w182:bool)
        n50 = Select(t="CheckRows", s=w182, f="Update: FilePath") -> (s? t:f=w177:string)
        n51 = call <vilib>:"Add State(s) to Queue__jki_lib_state_machine.vi"("State(s) in Front (\"\")"=w177, "State(s) in (\"\")"=w178) -> ("States Out"=w179:string)  [unwired: 13 in]
      }
      frame "SelectByBacode" {
        # "ResultTable\tValidColumnsNum\t25\t存储测试结果表格的有效数据列数。"
        # "Upload"
        n52 = call "Get Main.Parmeters.vi"("Main"="ResultTable", "VariableName"="ValidColumnsNum") -> ("DBL Value"=w229:dbl)  [unwired: 7 in, 6 out]
        n53 = To Long Integer(number=w229) -> (32bit integer=w228:i32)
        "32bit integer" <- w228
        n54 = Array Subset(array=w233, index=0, length=w228) -> (w224:string[])
        n55 = Index Array(array=w233, index #1=1 ("index"), index #2=2 ("index"), index #3=14 ("index")) -> (element #1=w222:string, element #2=w237:string, element #3=w226:string)
        n56 = Array Size(array=w224) -> (size(s)=→"size(s)":i32)
        n57 = Build Array(w222, w237, w226) -> (w256:string[])
        n58 = Build Array("0" ("element"), w252, "0" ("State(s) in (\"\")")) -> (w255:string[])
        n59 = call <userlib>:"SQL_Select From DB Table.vi"("DB Type"=T4."SQLite", "SelectedColumnsNameList"=w224, "ColumnsValue"=w255, "ColumnsNameList"=w256, "TableName"=w253) -> ("Select SQL CMD"=w241:string)  [unwired: 6 in]
        n60 = call-dynamic "SQL Execute.vi"("error in (no error)"=w246, "Return Data (T)"=TRUE, "Command Text"=w241, "HostDB in"=w251) -> ("error out"=w245:errorcluster, "Table Control"=w235:string[][], "HostDB out"=w250:refnum<class "SQLite.lvclass">)  [unwired: 3 in, 2 out]
        n61 = call <vilib>:"Add State(s) to Queue__jki_lib_state_machine.vi"("State(s) in Front (\"\")"=w240, "State(s) in (\"\")"=w241) -> ("States Out"=w242:string)  [unwired: 13 in]
        n62 = flat-sequence {
          tunnel: w235 -> [w260]
          tunnel: [w259] -> w234
          frame #0 {
            n63 = for {
              tunnel: w260 -> [w265] mode=indexing
              tunnel: [w264] -> w263 mode=indexing
              n64 = for {
                tunnel: w265 -> [w270] mode=indexing
                tunnel: [w266] -> w264
                i -> [w266]
                stop <- w267 stop-if-true
                n65 = String Length(string=w270) -> (length=w269:i32)
                n66 = Less?(x=w269, y=1) -> (x < y?=w267:bool)
              }
            }
            n67 = Array Max & Min(array=w263) -> (max value=w261:i32)  [unwired: 3 out]
            n68 = Array Subset(array=w260, index (col)=0 ("index"), length (col)=w261) -> (w259:string[][])  [unwired: 2 in]
          }
        }
        n69 = call <vilib>:"Add State(s) to Queue__jki_lib_state_machine.vi"("State(s) in (\"\")"=w247) -> ("States Out"=w248:string)  [unwired: 14 in]
        n70 = call <vilib>:"Add State(s) to Queue__jki_lib_state_machine.vi"("State(s) in (\"\")"=w243, "State(s) at Back (\"\")"=w242) -> ("States Out"=w244:string)  [unwired: 13 in]
      }
      frame "SelectByDatetime" {
        # "Upload"
        n71 = Get Date/Time In Seconds() -> (seconds since 1Jan1904=w281:timestamp)
        n72 = Index Array(array=w305, index #1=14 ("index"), index #2=0 ("index")) -> (element #1=w310:string, element #2=w276:string)
        n73 = Multiply(x=86400.0, y=15.0) -> (x*y=w287:dbl)
        n74 = To Double Precision Float(number=w281) -> (double precision float=w290:dbl)
        n75 = Build Array(w310) -> (w308:string[])
        n76 = Build Array("0" ("State(s) in (\"\")")) -> (w307:string[])
        n77 = Subtract(x=w290, y=w287) -> (x-y=w286:dbl)
        n78 = To Time Stamp(1:w286) -> (0:w282:timestamp)
        n79 = Format Date/Time String(time format string (%c)="%Y-%m-%d ", seconds (now)=w282) -> (date/time string=w285:string)  [unwired: 1 in]
        n80 = Format Date/Time String(time format string (%c)="%Y-%m-%d %H:%M:%S") -> (date/time string=w278:string)  [unwired: 2 in]
        n81 = Concatenate Strings(w285, "00:00:00" ("Numeric Text.Text 2")) -> (w279:string)
        n82 = call <userlib>:"SQL_Select From DB Table.vi"("DB Type"=T4."SQLite", "ColumnsValue"=w307, "ColumnsNameList"=w308, "TableName"=w304) -> ("Select SQL CMD"=w294:string)  [unwired: 7 in]
        n83 = call <userlib>:"Create Between DateTime.vi"("HaveWhere?"=FALSE, "End DateTime"=w278, "Start DateTime"=w279, "Column Name"=w276) -> ("Between DateTime"=w273:string)  [unwired: 7 in]
        n84 = Concatenate Strings(w294, w273) -> (w274:string)
        n85 = call-dynamic "SQL Execute.vi"("error in (no error)"=w299, "Command Text"=w274, "HostDB in"=w303) -> ("error out"=w298:errorcluster, "Table Control"=w272:string[][], "HostDB out"=w302:refnum<class "SQLite.lvclass">)  [unwired: 4 in, 2 out]
        n86 = flat-sequence {
          tunnel: w272 -> [w313]
          tunnel: [w312] -> w271
          frame #0 {
            n87 = for {
              tunnel: w313 -> [w318] mode=indexing
              tunnel: [w317] -> w316 mode=indexing
              n88 = for {
                tunnel: w318 -> [w323] mode=indexing
                tunnel: [w319] -> w317
                i -> [w319]
                stop <- w320 stop-if-true
                n89 = String Length(string=w323) -> (length=w322:i32)
                n90 = Less?(x=w322, y=1) -> (x < y?=w320:bool)
              }
            }
            n91 = Array Max & Min(array=w316) -> (max value=w314:i32)  [unwired: 3 out]
            n92 = Array Subset(array=w313, index (col)=0 ("index"), length (col)=w314) -> (w312:string[][])  [unwired: 2 in]
          }
        }
        n93 = call <vilib>:"Add State(s) to Queue__jki_lib_state_machine.vi"("State(s) in Front (\"\")"=w293, "State(s) in (\"\")"=w274) -> ("States Out"=w295:string)  [unwired: 13 in]
        n94 = call <vilib>:"Add State(s) to Queue__jki_lib_state_machine.vi"("State(s) in (\"\")"=w300) -> ("States Out"=w301:string)  [unwired: 14 in]
        n95 = call <vilib>:"Add State(s) to Queue__jki_lib_state_machine.vi"("State(s) in (\"\")"=w296, "State(s) at Back (\"\")"=w295) -> ("States Out"=w297:string)  [unwired: 13 in]
      }
      frame "Update" {
        n96 = Unbundle By Name(w347) -> ("Row Numbers"=w346:string)
        n97 = Index Array(array=w342, index=1) -> (element=w358:string)
        n98 = Index Array(array=w342, index #1=1 ("index")) -> (element #1=w341:string, element #2=w340:string, element #3=w339:string)  [unwired: 2 in]
        n99 = Build Array("0" ("element"), w354) -> (w336:string[])
        n100 = Build Array(w341, w340, w339) -> (w338:string[])
        n101 = Build Array(w358) -> (w356:string[])
        n102 = Build Array(w346) -> (w345:string[])
        n103 = call <userlib>:"Build string_ColumnsName=ColumnsValue_Where and.vi"("DB Type"=T4."SQLite", "ColumnsValue"=w336, "Check ASCII?"=FALSE, "ColumnsNameList"=w338) -> ("ColumnName='ColumnValue'"=w344:string)  [unwired: 7 in]
        n104 = call <userlib>:"SQL_Update DB Table.vi"("where name='value'"=w344, "ColumnsValue"=w345, "ColumnsNameList"=w356, "TableName"=w355) -> ("Update CMD"=w326:string)  [unwired: 7 in]
        n105 = call-dynamic "SQL Execute.vi"("error in (no error)"=w350, "Return Data (T)"=FALSE, "Command Text"=w326, "HostDB in"=w353) -> ("error out"=w333:errorcluster, "HostDB out"=w352:refnum<class "SQLite.lvclass">)  [unwired: 3 in, 3 out]
        n106 = Select(t="", s=w333, f="Insert") -> (s? t:f=w331:string)
        n107 = call <vilib>:"Add State(s) to Queue__jki_lib_state_machine.vi"("State(s) in Front (\"\")"=w325, "State(s) in (\"\")"=w326) -> ("States Out"=w327:string)  [unwired: 13 in]
        n108 = call <vilib>:"Add State(s) to Queue__jki_lib_state_machine.vi"("State(s) in Front (\"\")"=w331, "State(s) in (\"\")"=w348) -> ("States Out"=w349:string)  [unwired: 13 in]
        n109 = call <vilib>:"Add State(s) to Queue__jki_lib_state_machine.vi"("State(s) in (\"\")"=w328, "State(s) at Back (\"\")"=w327) -> ("States Out"=w329:string)  [unwired: 13 in]
      }
      frame "Update-UploadColumn" {
        n110 = Unbundle By Name(w378) -> ()  [unwired: 1 out]
        n111 = Index Array(array=w374, index=14) -> (element=w389:string)
        "element" <- w389
        n112 = Index Array(array=w374, index #1=1 ("index")) -> (element #1=w373:string, element #2=w372:string)  [unwired: 1 in]
        n113 = Build Array(w360, w385) -> (w370:string[])
        n114 = Build Array(w373, w372) -> (w371:string[])
        n115 = Build Array(w389) -> (w387:string[])
        n116 = Build Array("1") -> (w377:string[])
        n117 = call <userlib>:"Build string_ColumnsName=ColumnsValue_Where and.vi"("DB Type"=T4."SQLite", "ColumnsValue"=w370, "Check ASCII?"=FALSE, "ColumnsNameList"=w371) -> ("ColumnName='ColumnValue'"=w376:string)  [unwired: 7 in]
        n118 = call <userlib>:"SQL_Update DB Table.vi"("where name='value'"=w376, "ColumnsValue"=w377, "ColumnsNameList"=w387, "TableName"=w386) -> ("Update CMD"=w364:string)  [unwired: 7 in]
        "Update CMD" <- w364
        n119 = call-dynamic "SQL Execute.vi"("error in (no error)"=w381, "Return Data (T)"=FALSE, "Command Text"=w364, "HostDB in"=w384) -> ("HostDB out"=w383:refnum<class "SQLite.lvclass">)  [unwired: 3 in, 4 out]
        n120 = call <vilib>:"Add State(s) to Queue__jki_lib_state_machine.vi"("State(s) in Front (\"\")"=w363, "State(s) in (\"\")"=w364) -> ("States Out"=w365:string)  [unwired: 13 in]
        n121 = call <vilib>:"Add State(s) to Queue__jki_lib_state_machine.vi"("State(s) in (\"\")"=w379) -> ("States Out"=w380:string)  [unwired: 14 in]
        n122 = call <vilib>:"Add State(s) to Queue__jki_lib_state_machine.vi"("State(s) in (\"\")"=w366, "State(s) at Back (\"\")"=w365) -> ("States Out"=w367:string)  [unwired: 13 in]
      }
      frame "Update: FilePath" {
        n123 = Unbundle By Name(w405) -> ("Results Folder path"=w406:path, "RowNum"=w399:i32)  [unwired: 1 out]
        n124 = case shown="2.." w399 {
          selector: w399 -> [_ w437 _]
          tunnel: w408 -> [w435 w440 w442]
          tunnel: [w435 w439 w441] -> w409
          frame Default {
          }
          frame 2.. {
            n125 = Number To Decimal String(number=w437) -> (decimal integer string=w436:string)  [unwired: 1 in]
            n126 = Concatenate Strings(w440, "_" ("string"), w436) -> (w439:string)
          }
          frame 0 {
            n127 = Concatenate Strings(w442) -> (w441:string)
          }
        }
        n128 = call "Get Main.Parmeters.vi"("VariableName"="ResultsFileFormat") -> ("Value"=w395:string)  [unwired: 8 in, 6 out]
        n129 = Empty String/Path?(string/path=w409) -> (empty?=w413:bool)
        n130 = Format Date/Time String(time format string (%c)=w407) -> (date/time string=w412:string)  [unwired: 2 in]
        n131 = Select(t=w412, s=w413, f=w409) -> (s? t:f=w410:string)
        n132 = Concatenate Strings(w410, w395) -> (w411:string)
        n133 = Build Path(base path=w406, name or relative path=w411) -> (appended path=w397:path)
        n134 = Path To String(path=w397) -> (string=w394:string)
        n135 = Index Array(array=w422, index=13) -> (element=w433:string)
        n136 = Index Array(array=w422, index #1=1 ("index")) -> (element #1=w421:string, element #2=w420:string, element #3=w419:string)  [unwired: 2 in]
        n137 = Build Array("0" ("element"), w408) -> (w416:string[])
        n138 = Build Array(w421, w420, w419) -> (w418:string[])
        n139 = Build Array(w433) -> (w431:string[])
        n140 = Build Array(w394) -> (w425:string[])
        n141 = call <userlib>:"Build string_ColumnsName=ColumnsValue_Where and.vi"("DB Type"=T4."SQLite", "ColumnsValue"=w416, "Check ASCII?"=FALSE, "ColumnsNameList"=w418) -> ("ColumnName='ColumnValue'"=w424:string)  [unwired: 7 in]
        n142 = call <userlib>:"SQL_Update DB Table.vi"("where name='value'"=w424, "ColumnsValue"=w425, "ColumnsNameList"=w431, "TableName"=w430) -> ("Update CMD"=w401:string)  [unwired: 7 in]
        n143 = call-dynamic "SQL Execute.vi"("error in (no error)"=w393, "Command Text"=w401, "HostDB in"=w429) -> ("error out"=w391:errorcluster, "HostDB out"=w428:refnum<class "SQLite.lvclass">)  [unwired: 4 in, 3 out]
        n144 = call <vilib>:"Add State(s) to Queue__jki_lib_state_machine.vi"("State(s) in Front (\"\")"=w400, "State(s) in (\"\")"=w401) -> ("States Out"=w402:string)  [unwired: 13 in]
        n145 = Bundle By Name(cluster=w405, "ResultFilePath"=w397) -> (w398:T2)
        n146 = call <vilib>:"Add State(s) to Queue__jki_lib_state_machine.vi"("State(s) in (\"\")"=w403, "State(s) at Back (\"\")"=w402) -> ("States Out"=w404:string)  [unwired: 13 in]
        n147 = call <vilib>:"Add State(s) to Queue__jki_lib_state_machine.vi"("State(s) in (\"\")"=w426) -> ("States Out"=w427:string)  [unwired: 14 in]
      }
      frame "State3" {
      }
    }
  }
  "CMD" <- w15
  n148 = Random Number (0-1)() -> (number: 0 to 1=→"number (0 to 1)":dbl)
  n149 = call-dynamic "Close Connection.vi"("HostDB in"=w23) -> ("error out"=w29:errorcluster)  [unwired: 9 in, 1 out]
  n150 = disable-structure shown="Disabled" {
    disable-tunnel: w10 -> [w450 _]
    frame Disabled {
      "Table Control" <- w450
    }
    frame Enabled {
    }
  }
  n151 = Merge Errors(w29, w21) -> (→"error out":errorcluster)
  n152 = Array Subset(array=w10, index (row)=0 ("index"), length (row)=3 ("length")) -> (w6:string[][])  [unwired: 2 in]
  n153 = Index Array(array=w6, index (col)=13 ("disabled index (col)")) -> (element=→"File Paht":string[])  [unwired: 1 in]
  n154 = Delete From Array(array=w6, length=1, index (col)=0 ("disabled index (col)")) -> (array with subset deleted=→"30 rows":string[][])  [unwired: 1 in, 1 out]
